vi "ReportEnd.vi"(6 "文件重命名":bool, 8 "error in (no error)":errorcluster caption="错误输入（无错误）", 10 "文件名称":string, 11 "report in":refnum<class "NI_report.lvclass"> caption="报表输入") -> (0 "error out":errorcluster caption="错误输出")   [LabVIEW 2020]
uses:
  <vilib>/Utility/NIReport.llb/NI_report.lvclass
  Global_Variable/Global.vi
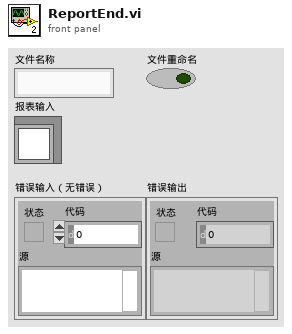
[diagram p1: front panel]
types:
  T1 = cluster{"Italic":enum16{"Italic Unchanged", "Italic On", "Italic Off"}, "Strike Through":enum16{"Strike Through Unchanged", "Strike Through On", "Strike Through Off"}, "Underline":enum16{"Underline Unchanged", "Underline On", "Underline Off"}, "Bold":enum16{"Bold Unchanged", "Bold On", "Bold Off"}}
  T2 = cluster{"Charset (-1)":i16, "Weight (-1)":i16, "Name":string, "Size":string}
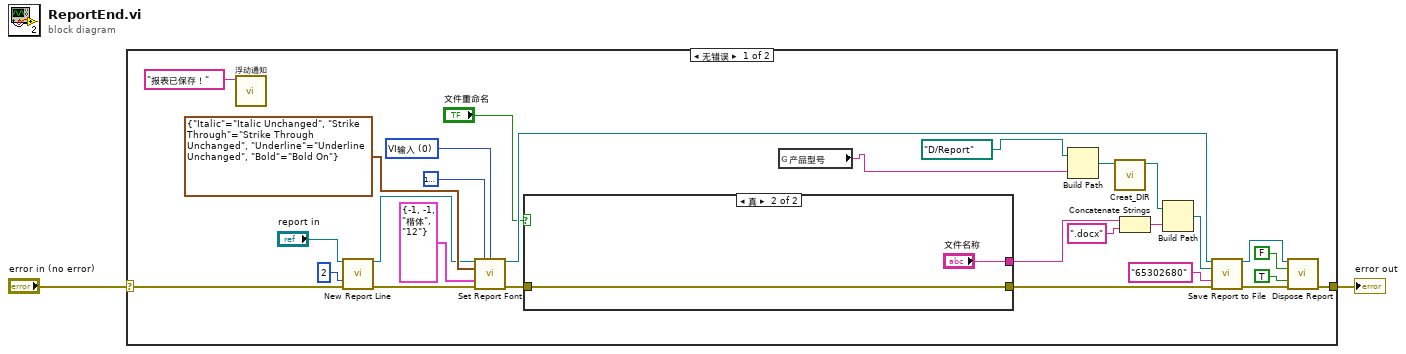
[diagram p0: block diagram]
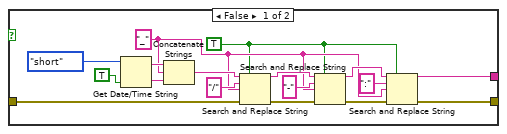
[diagram p2: hidden frame]
diagram:
  n1 = case shown="无错误" "error in (no error)" {
    selector: "error in (no error)" -> [w15 w50]
    tunnel: [w14 w50] -> w1
    frame No Error {
      w25 = u16 0 items=["VI输入", "字体对话框"] ("font settings source")
      n2 = call "浮动通知.vi"("通知内容"="报表已保存！" ("Status")) -> ()  [unwired: 11 in]
      n3 = call-dynamic "New Report Line.vi"("report in"="report in", "number of lines (1)"=2, "error in (no error)"=w15) -> ("report out"=w22:refnum<class "NI_report.lvclass">, "error out"=w21:errorcluster)  [unwired: 11 in]
      n4 = call-dynamic "Set Report Font.vi"("report in"=w22, "text color (unchanged)"=u32 16777224, "font settings source (VI Inputs)"=w25, "text options"=T1 {"Italic"=enum."Italic Unchanged", "Strike Through"=enum."Strike Through Unchanged", "Underline"=enum."Underline Unchanged", "Bold"=enum."Bold On"}, "font settings"=T2 {"Charset (-1)"=-1, "Weight (-1)"=-1, "Name"="楷体", "Size"="12"}, "error in (no error)"=w21) -> ("report out"=w18:refnum<class "NI_report.lvclass">, "error out"=w17:errorcluster)  [unwired: 7 in, 1 out]
      n5 = case shown="真" "文件重命名" {
        tunnel: [w42 "文件名称"] -> w12
        tunnel: w17 -> [w34 w49]
        tunnel: [w31 w49] -> w16
        frame False {
          w36 = TRUE ("替换全部？(F)")
          w37 = "_" ("替换字符串(\"\")")
          n6 = Get Date/Time String(date format (0)=enum16{"short", "long", "abbreviated"}."short" ("日期格式(0)"), want seconds? (F)=TRUE ("需要秒？(F)")) -> (date string=w47:string, time string=w43:string)  [unwired: 1 in]
          n7 = Concatenate Strings(w47, w37, w43) -> (w40:string)
          n8 = Search and Replace String(replace all?=w36, input string=w40, search string="/" ("搜索字符串"), replace string=w37, error in=w34) -> (result string=w39:string, error out=w33:errorcluster)  [unwired: 3 in, 2 out]
          n9 = Search and Replace String(replace all?=w36, input string=w39, search string="-" ("搜索字符串"), replace string=w37, error in=w33) -> (result string=w45:string, error out=w32:errorcluster)  [unwired: 3 in, 2 out]
          n10 = Search and Replace String(replace all?=w36, input string=w45, search string=":" ("搜索字符串"), replace string=w37, error in=w32) -> (result string=w42:string, error out=w31:errorcluster)  [unwired: 3 in, 2 out]
        }
        frame True {
        }
      }
      n11 = global read "Global.vi" "产品型号"() -> (w3:string)
      n12 = Build Path(base path=path "D:/Report" ("report file path"), name or relative path=w3) -> (appended path=w6:path)
      n13 = call "Creat_DIR.vi"("path"=w6) -> ("created path"=w5:path)  [unwired: 10 in]
      n14 = Concatenate Strings(w12, ".docx" ("字符串")) -> (w11:string)
      n15 = Build Path(base path=w5, name or relative path=w11) -> (appended path=w4:path)
      n16 = call-dynamic "Save Report to File.vi"("report in"=w18, "report file path"=w4, "password (\"\")"="65302680" ("password (\"\")"), "error in (no error)"=w16) -> ("report out"=w30:refnum<class "NI_report.lvclass">, "error out"=w29:errorcluster)  [unwired: 10 in]
      n17 = call-dynamic "Dispose Report.vi"("report in"=w30, "wait until printing completed? (T)"=FALSE, "save changes? (F)"=TRUE, "error in (no error)"=w29) -> ("error out"=w14:errorcluster)  [unwired: 11 in]
    }
    frame Error {
    }
  }
  "error out" <- w1
